vi "netstat.vi"(8 "error in (no error)":errorcluster) -> (0 "error out":errorcluster, 3 "netstat":T1(array[cluster]))   [LabVIEW 2025]
doc: "This VI queries the network stack and list the state of each active network connection.\n\nCreated By: Ryan Pacini"
panel:
  out "standard output":string
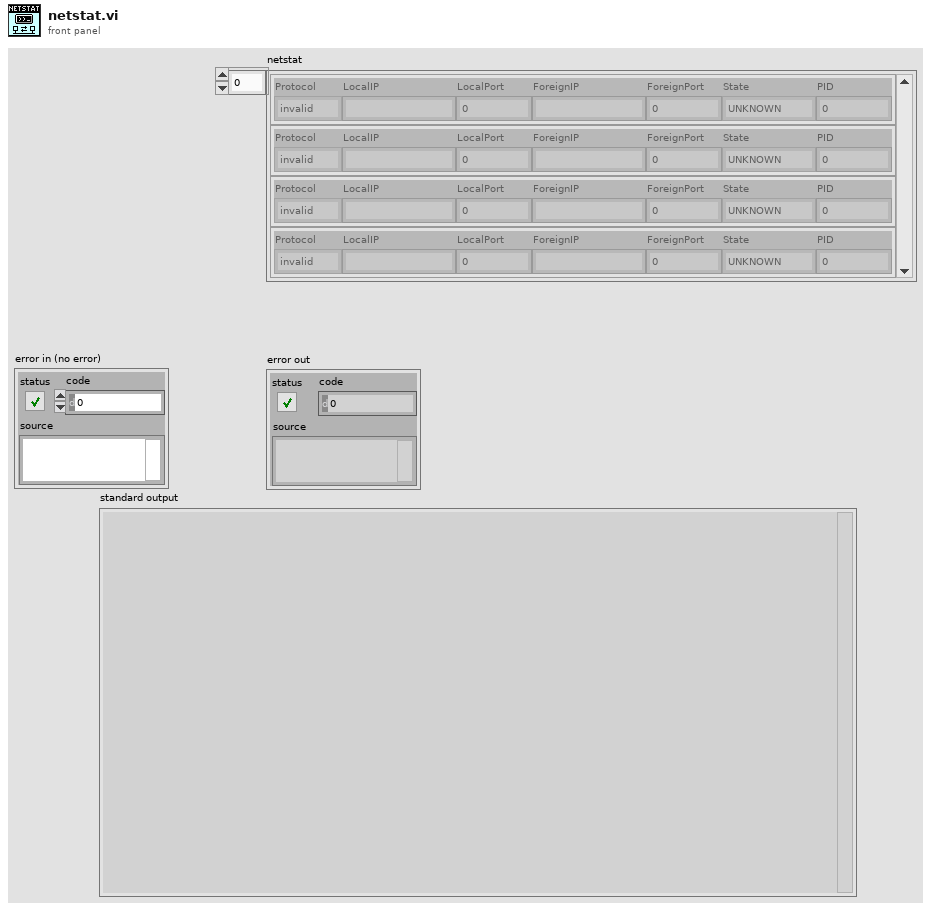
[diagram p1: front panel]
types:
  T1 = cluster{"Protocol":enum16{"invalid", "tcp", "udp", "icmp", "ip", "tcpv6", "udpv6", "icmpv6", "ipv6"}, "LocalIP":string, "LocalPort":u16, "ForeignIP":string, "ForeignPort":u16, "State":enum8{"UNKNOWN", "LISTEN", "ESTABLISHED", "SYN_SENT", "SYN_RECV", "LAST_ACK", "CLOSE_WAIT", "TIME_WAIT", "CLOSED", "CLOSING", "FIN_WAIT1", "FIN_WAIT2"}, "PID":u16}[]
  T2 = enum16{"invalid", "tcp", "udp", "icmp", "ip", "tcpv6", "udpv6", "icmpv6", "ipv6"}
  T3 = cluster{"Protocol":enum16{"invalid", "tcp", "udp", "icmp", "ip", "tcpv6", "udpv6", "icmpv6", "ipv6"}, "LocalIP":string, "LocalPort":u16, "ForeignIP":string, "ForeignPort":u16, "State":enum8{"UNKNOWN", "LISTEN", "ESTABLISHED", "SYN_SENT", "SYN_RECV", "LAST_ACK", "CLOSE_WAIT", "TIME_WAIT", "CLOSED", "CLOSING", "FIN_WAIT1", "FIN_WAIT2"}, "PID":u16}
  T4 = enum8{"UNKNOWN", "LISTEN", "ESTABLISHED", "SYN_SENT", "SYN_RECV", "LAST_ACK", "CLOSE_WAIT", "TIME_WAIT", "CLOSED", "CLOSING", "FIN_WAIT1", "FIN_WAIT2"}
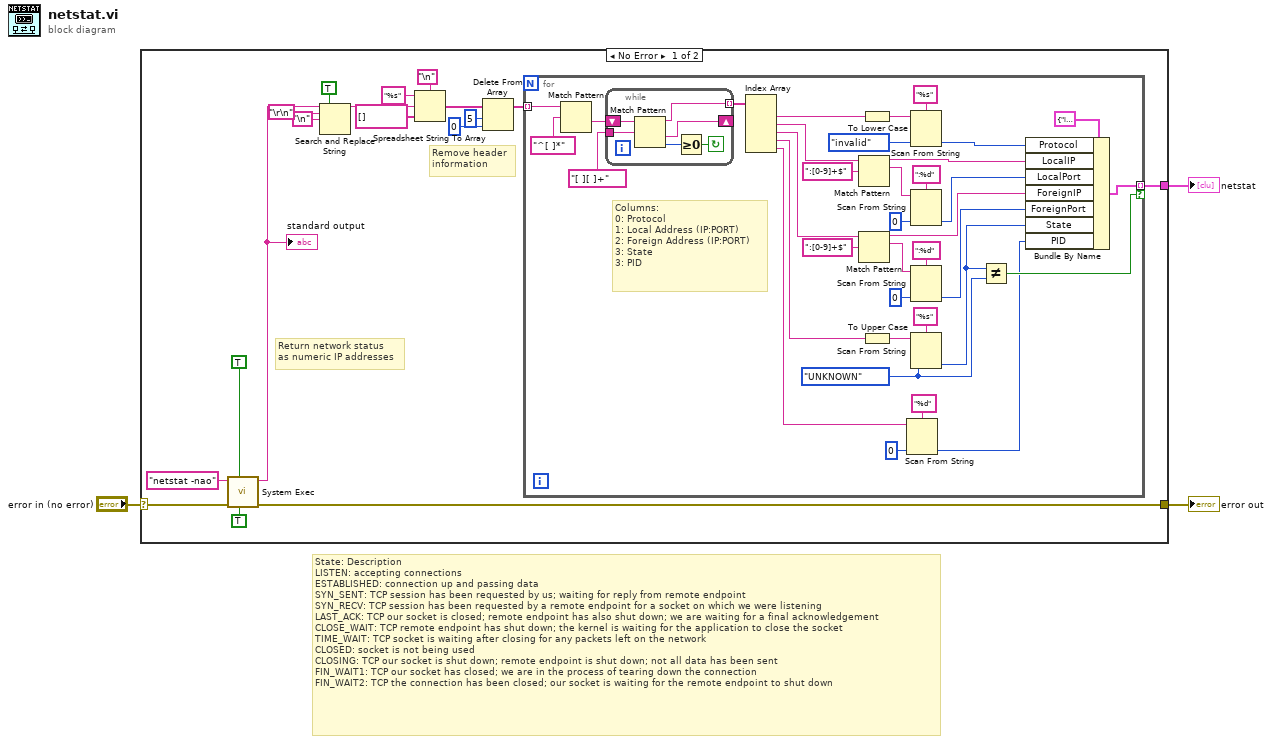
[diagram p0: block diagram]
diagram:
  # "State: Description\nLISTEN: accepting connections\nESTABLISHED: connection up and passing data\nSYN_SENT: TCP session has been requested by us; waiting for reply from remote endpoint\nSYN_RECV: TCP session has been requested by a remote endpoint for a socket on which we were listening\nLAST_ACK: TCP our socket is closed; remote endpoint has also shut down; we are waiting for a final acknowledgement\nCLOSE_WAIT: TCP remote endpoint has shut down; the kernel is waiting for the application to close the socket\nTIME_WAIT: TCP socket is waiting after closing for any packets left on the network\nCLOSED: socket is not being used\nCLOSING: TCP our socket is shut down; remote endpoint is shut down; not all data has been sent\nFIN_WAIT1: TCP our socket has closed; we are in the process of tearing down the connection\nFIN_WAIT2: TCP the connection has been closed; our socket is waiting for the remote endpoint to shut down"
  n1 = case shown="No Error" "error in (no error)" {
    selector: "error in (no error)" -> [w19 w64]
    tunnel: [w18 w64] -> w2
    tunnel: [w4 _] -> w1
    frame No Error {
      # "Return network status\nas numeric IP addresses"
      # "Remove header\ninformation"
      n2 = call <vilib>:"System Exec.vi"("run minimized? (F)"=TRUE, "wait until completion? (T)"=TRUE, "error in (no error)"=w19, "command line"="netstat -nao") -> ("error out"=w18:errorcluster, "standard output"=w16:string)  [unwired: 4 in, 2 out]
      "standard output" <- w16
      n3 = Search and Replace String(replace all?=TRUE ("replace all? (F)"), input string=w16, search string="\r\n" ("End of Line Constant"), replace string="\n" ("Line Feed Constant")) -> (result string=w12:string)  [unwired: 4 in, 3 out]
      n4 = Spreadsheet String To Array(delimiter (Tab)="\n", format string="%s", spreadsheet string=w12, array type (2D Dbl)=string[] []) -> (array=w8:string[])
      n5 = Delete From Array(array=w8, length=5, index=0) -> (array with subset deleted=w7:string[])  [unwired: 1 out]
      n6 = for {
        tunnel: w7 -> [w50] mode=indexing
        tunnel: [w51] -> w4 mode=indexing if=w31
        w29 = T4."UNKNOWN" ("State")
        # "Columns:\n0: Protocol\n1: Local Address (IP:PORT)\n2: Foreign Address (IP:PORT)\n3: State\n3: PID"
        n7 = Match Pattern(string=w50, regular expression="^[ ]*") -> (after substring=w49:string)  [unwired: 1 in, 3 out]
        n8 = while {
          shift-right: [w61] -> _
          shift-left: w49 -> [w62]
          tunnel: [w60] -> w56 mode=indexing
          tunnel: "[ ][ ]+" ("regular expression") -> [w58]
          stop <- w59 continue-if-true
          n9 = Match Pattern(string=w62, regular expression=w58) -> (before substring=w60:string, after substring=w61:string, offset past match=w63:i32)  [unwired: 1 in, 1 out]
          n10 = Greater Or Equal To 0?(x=w63) -> (x >= 0?=w59:bool)
        }
        n11 = Index Array(array=w56) -> (element #1=w54:string, element #2=w47:string, element #3=w40:string, element #4=w37:string, element #5=w22:string)  [unwired: 5 in]
        n12 = Match Pattern(string=w47, regular expression=":[0-9]+$") -> (before substring=w28:string, match substring=w34:string)  [unwired: 1 in, 2 out]
        n13 = Match Pattern(string=w40, regular expression=":[0-9]+$") -> (before substring=w39:string, match substring=w35:string)  [unwired: 1 in, 2 out]
        n14 = To Lower Case(string=w54) -> (all lower case string=w52:string)
        n15 = To Upper Case(1:w37) -> (0:w36:string)
        n16 = Scan From String(format string="%d", input string=w22, default 1=u16 0 ("default value 1")) -> (output 1=w23:u16)  [unwired: 2 in, 3 out]
        n17 = Scan From String(format string="%s", input string=w52, default 1=T2."invalid" ("Protocol")) -> (output 1=w33:T2)  [unwired: 2 in, 3 out]
        n18 = Scan From String(format string=":%d", input string=w34, default 1=u16 0 ("default value 1")) -> (output 1=w27:u16)  [unwired: 2 in, 3 out]
        n19 = Scan From String(format string=":%d", input string=w35, default 1=u16 0 ("default value 1")) -> (output 1=w26:u16)  [unwired: 2 in, 3 out]
        n20 = Scan From String(format string="%s", input string=w36, default 1=w29) -> (output 1=w30:T4)  [unwired: 2 in, 3 out]
        n21 = Not Equal?(x=w30, y=w29) -> (x != y?=w31:bool)
        n22 = Bundle By Name(cluster=T3 {"Protocol"=enum."invalid", "LocalIP"="", "LocalPort"=0, "ForeignIP"="", "ForeignPort"=0, "State"=enum."UNKNOWN", "PID"=0} ("netstat"), "Protocol"=w33, "LocalIP"=w28, "LocalPort"=w27, "ForeignIP"=w39, "ForeignPort"=w26, "State"=w30, "PID"=w23) -> (w51:T3)
      }
    }
    frame Error {
    }
  }
  "error out" <- w2
  "netstat" <- w1
